vi "SoundSensor Example.vi"() -> ()   [LabVIEW 2012, in "Phidget Sound Sensor.lvlib"]
uses:
  <instrlib>/Phidgets/Phidget Sound Sensor/Phidget Sound Sensor.lvlib
  <instrlib>/Phidgets/Phidget Sound Sensor/Public/SoundSensorStart.vi
  <instrlib>/Phidgets/Phidget Sound Sensor/Public/SoundSensorClose.vi
  <instrlib>/Phidgets/Phidget Common/Phidget Common.lvlib
panel:
  out "Octaves":dbl[](array[numeric])
  out "dBA":dbl
  out "dBC":dbl
  out "dB":dbl caption="Illuminance"
  out "error out":errorcluster
  in  "error in (no error)":errorcluster
  in  "Device Info":T1={"Serial Number"=-1, "Channel"=0, "Port"=0}
  out "Attached?":bool
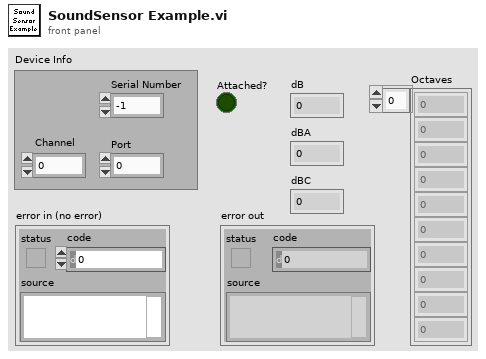
[diagram p1: front panel]
types:
  T1 = cluster{"Serial Number":i32, "Channel":i32, "Port":i32}
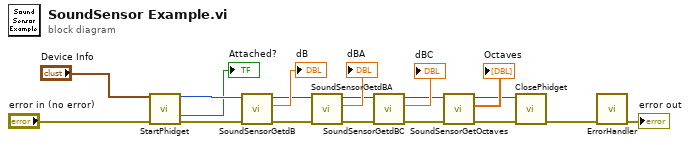
[diagram p0: block diagram]
diagram:
  n1 = call-poly <instrlib>:"StartPhidget.vi"("Device Info"="Device Info", "error in (no error)"="error in (no error)") -> ("Phidget ID"=w19:u64, "Attached?"=→"Attached?":bool, "error out"=w18:errorcluster)  [unwired: 10 in, 1 out]
  n2 = call <instrlib>:"SoundSensorGetdB.vi"("error in (no error)"=w18, "Device In"=w19) -> ("error out"=w7:errorcluster, "dB"=→"dB":dbl, "Device Out"=w9:u64)  [unwired: 6 in]
  n3 = call <instrlib>:"SoundSensorGetdBA.vi"("error in (no error)"=w7, "Device In"=w9) -> ("error out"=w6:errorcluster, "dBA"=→"dBA":dbl, "Device Out"=w8:u64)  [unwired: 6 in]
  n4 = call <instrlib>:"SoundSensorGetdBC.vi"("error in (no error)"=w6, "Device In"=w8) -> ("error out"=w4:errorcluster, "dBC"=→"dBC":dbl, "Device Out"=w5:u64)  [unwired: 6 in]
  n5 = call <instrlib>:"SoundSensorGetOctaves.vi"("error in (no error)"=w4, "Device In"=w5) -> ("error out"=w3:errorcluster, "Octaves"=→"Octaves":dbl[], "Device Out"=w1:u64)  [unwired: 6 in]
  n6 = call-poly <instrlib>:"ClosePhidget.vi"("error in"=w3, "Device In"=w1) -> ("error out"=w14:errorcluster)  [unwired: 9 in]
  n7 = call <instrlib>:"ErrorHandler.vi"("error in"=w14) -> ("error out"=→"error out":errorcluster)  [unwired: 9 in, 1 out]
